vi "FTW-Publisher-Socket Publisher.vi"(1 "Endpoint":refnum<class "FTW-Endpoint.lvclass">, 2 "Message Handler":refnum<user-event>) -> ()   [LabVIEW 2013, in "FTW-Publisher.lvclass"]
uses:
  FTW-Publisher.lvclass
  Message/Base/FTW-Message.lvclass
  Endpoint/FTW-Endpoint.lvclass
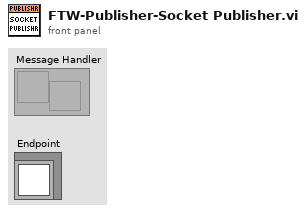
[diagram p1: front panel]
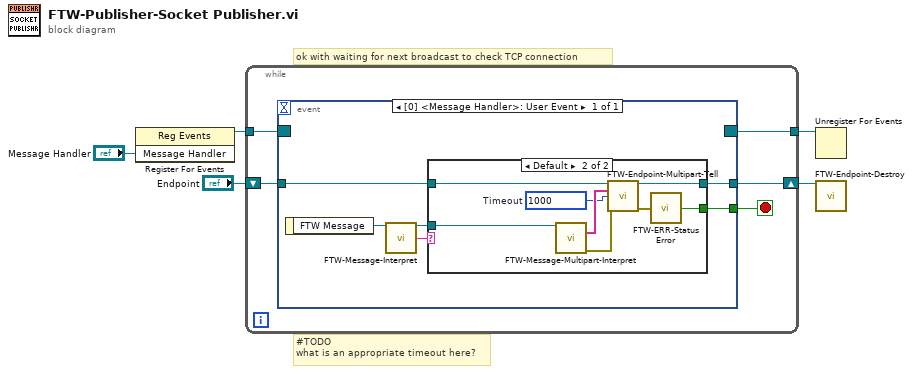
[diagram p0: block diagram]
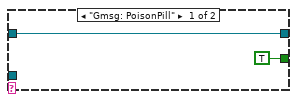
[diagram p2: hidden frame]
diagram:
  # "#TODO\nwhat is an appropriate timeout here?"
  # "ok with waiting for next broadcast to check TCP connection"
  n1 = register-events("Message Handler") -> (reference out=w1:refnum<event-registration>)  [unwired: 2 in, 1 out]
  n2 = while {
    tunnel: w1 -> [w10]
    tunnel: [w7] -> w4
    shift-right: [w6] -> w5
    shift-left: "Endpoint" -> [w9]
    stop <- w8 stop-if-true
    n3 = event shown="[0] <Message Handler>: User Event" {
      selector: w10 -> [_]
      dyn-events: [_] -> w7
      timeout: _ -> [_]
      tunnel: w9 -> [w16]
      tunnel: [w14] -> w8
      tunnel: [w15] -> w6
      event User Event {
        n4 = event-data() -> ("FTW Message"=w13:refnum<class "FTW-Message.lvclass">)  [unwired: 1 in]
        n5 = call-dynamic "FTW-Message-Interpret.vi"("FTW Message"=w13) -> ("FTW Message out"=w12:refnum<class "FTW-Message.lvclass">, "Message Header"=w11:string)  [unwired: 10 in, 3 out]
        n6 = case shown="Default" w11 {
          tunnel: w16 -> [w18 w26]
          tunnel: [w18 w24] -> w15
          tunnel: [TRUE ("status") w23] -> w14
          tunnel: w12 -> [_ w22]
          frame "Gmsg: PoisonPill" {
          }
          frame Default {
            w19 = 1000  # Timeout
            n7 = call-dynamic "FTW-Message-Multipart-Interpret.vi"("FTW Message"=w22) -> ("Message Parts"=w20:string[], "error out"=w21:errorcluster)  [unwired: 12 in, 1 out]
            n8 = call-dynamic "FTW-Endpoint-Multipart-Tell.vi"("FTW Endpoint"=w26, "Multipart Message"=w20, "Timeout"=w19, "error in"=w21) -> ("FTW Endpoint out"=w24:refnum<class "FTW-Endpoint.lvclass">, "error out"=w25:errorcluster)  [unwired: 9 in, 1 out]
            n9 = call "FTW-ERR-StatusError.vi"("error to check"=w25) -> ("Error?"=w23:bool)
          }
        }
      }
    }
  }
  n10 = Unregister For Events(event registration refnum=w4) -> ()  [unwired: 1 in, 1 out]
  n11 = call-dynamic "FTW-Endpoint-Destroy.vi"("FTW Endpoint"=w5) -> ()  [unwired: 14 in, 1 out]
